vi "Unflatten Value.vi"(8 "Error In":errorcluster, 10 "Value":string, 11 "Int In":refnum<class "Int.lvclass">) -> (0 "Error Out":errorcluster, 3 "Int Out":refnum<class "Int.lvclass">)   [LabVIEW 2020, in "NI_VIAnCFGDataStructure.lvlib" / "Int.lvclass"]
uses:
  <vilib>/addons/analyzer/VIAnCFGDataStructure/Data Types/Int/Int.lvclass
  <vilib>/addons/analyzer/VIAnCFGDataStructure/Data Types/Int/Int.lvclass/Int.ctl
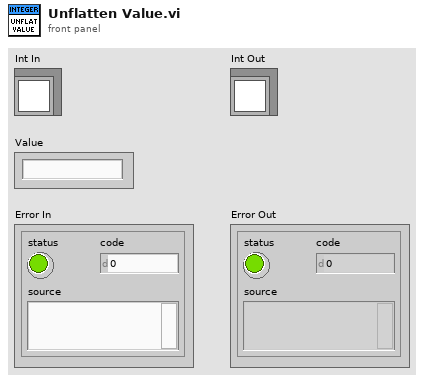
[diagram p1: front panel]
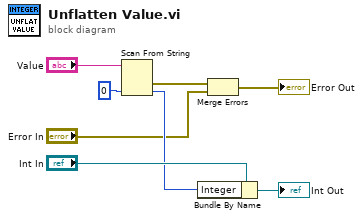
[diagram p0: block diagram]
diagram:
  n1 = Scan From String(input string="Value", default 1=i64 0 ("default value 1")) -> (error out=w3:errorcluster, output 1=w4:i64)  [unwired: 3 in, 2 out]
  n2 = Bundle By Name(cluster="Int In", "Integer"=w4) -> (→"Int Out":refnum<class "Int.lvclass">)
  n3 = Merge Errors(w3, "Error In") -> (→"Error Out":errorcluster)
